vi "Obtain Message Queue.vi"(8 "error in (no error)":errorcluster) -> (0 "error out":errorcluster, 3 "Message Queue":refnum<class "Message Queue.lvclass">)   [LabVIEW 2017, in "Actor Framework.lvlib" / "Message Queue.lvclass"]
doc: "(<B>Filename</B>: Actor Framework.lvlib:Message Queue.lvclass:Obtain Message Queue.vi)\n\nObtains the reference to the message queue that the caller uses to communicate with the top-level actor."
uses:
  Message Queue.lvclass
  Message Enqueuer/Message Enqueuer.lvclass/Message Enqueuer.ctl
  Message Dequeuer/Message Dequeuer.lvclass/Message Dequeuer.ctl
  Message Queue.lvclass/Message Queue.ctl
  Message Enqueuer/Message Enqueuer.lvclass
  Message Dequeuer/Message Dequeuer.lvclass
  Message Priority Queue/Message Priority Queue.lvclass
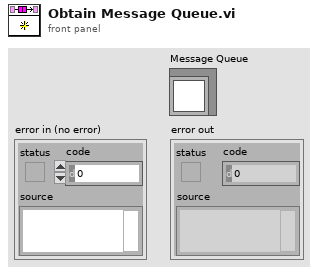
[diagram p1: front panel]
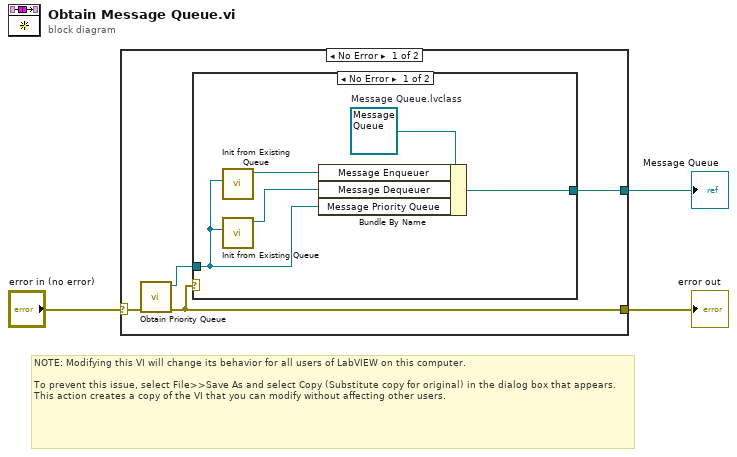
[diagram p0: block diagram]
diagram:
  # "NOTE: Modifying this VI will change its behavior for all users of LabVIEW on this computer.\n\nTo prevent this issue, select File>>Save As and select Copy (Substitute copy for original) in the dialog box that appears. This action creates a copy of the VI that you can modify without affecting other users."
  n1 = case shown="No Error" "error in (no error)" {
    selector: "error in (no error)" -> [w7 w13]
    tunnel: [w5 w13] -> w2
    tunnel: [w6 _] -> w1
    frame No Error {
      n2 = call "Obtain Priority Queue.vi"("error in (no error)"=w7) -> ("error out"=w5:errorcluster, "Priority Queue"=w4:refnum<class "Message Priority Queue.lvclass">)  [unwired: 9 in]
      n3 = case shown="No Error" w5 {
        tunnel: [w11 _] -> w6
        tunnel: w4 -> [w8 _]
        frame No Error {
          w12 = refnum<class "Message Queue.lvclass"> refnum  # Message Queue.lvclass
          n4 = call "Init from Existing Queue.vi"("Priority Queue"=w8) -> ("Message Enqueuer"=w10:refnum<class "Message Enqueuer.lvclass">)  [unwired: 10 in]
          n5 = call "Init from Existing Queue.vi"("Priority Queue"=w8) -> ("Message Dequeuer"=w9:refnum<class "Message Dequeuer.lvclass">)  [unwired: 10 in]
          n6 = Bundle By Name(cluster=w12, "Message Enqueuer"=w10, "Message Dequeuer"=w9, "Message Priority Queue"=w8) -> (w11:refnum<class "Message Queue.lvclass">)
        }
        frame Error {
        }
      }
    }
    frame Error {
    }
  }
  "error out" <- w2
  "Message Queue" <- w1
